vi "InputDriveCommands.vi"(11 "All Joysticks":T3) -> (3 "Drive Command Inputs":T1)   [LabVIEW 2012]
uses:
  Input_All_Joysticks.ctl
  Input_Single_Joystick.ctl
  <vilib>/Rock Robotics/WPI/Joystick/WPI_JoystickButtonState.ctl
  Kinect/KinectInputs.ctl
  Input_Commands_Drive.ctl
panel:
  in  "Kinect Inputs":T2
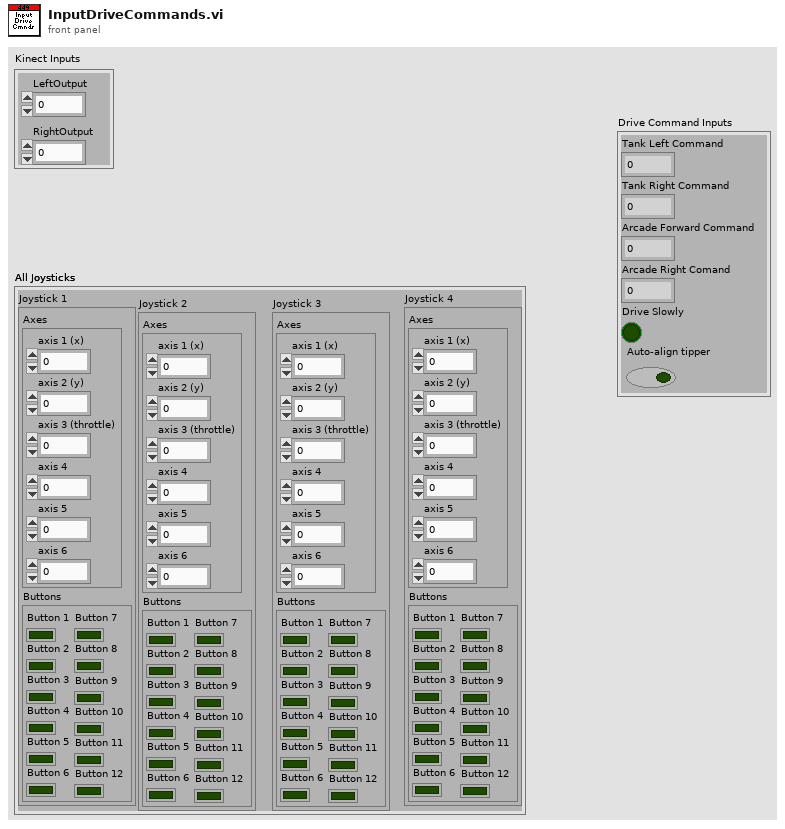
[diagram p1: front panel]
types:
  T1 = typedef "Input_Commands_Drive.ctl" = cluster{"Tank Left Command":dbl, "Tank Right Command":dbl, "Arcade Forward Command":dbl, "Arcade Right Comand":dbl, "Drive Slowly":bool, "Auto-align tipper":bool}
  T2 = typedef "KinectInputs.ctl" = cluster{"LeftOutput":dbl, "RightOutput":dbl}
  T3 = typedef "Input_All_Joysticks.ctl" = cluster{"Joystick 1":T4, "Joystick 2":T4, "Joystick 3":T4, "Joystick 4":T4}
  T4 = typedef "Input_Single_Joystick.ctl" = cluster{"Axes":cluster{"axis 1 (x)":dbl, "axis 2 (y)":dbl, "axis 3 (throttle)":dbl, "axis 4":dbl, "axis 5":dbl, "axis 6":dbl}, "Buttons":T5}
  T5 = typedef "WPI_JoystickButtonState.ctl" = cluster{"Button 1":bool, "Button 2":bool, "Button 3":bool, "Button 4":bool, "Button 5":bool, "Button 6":bool, "Button 7":bool, "Button 8":bool, "Button 9":bool, "Button 10":bool, "Button 11":bool, "Button 12":bool}
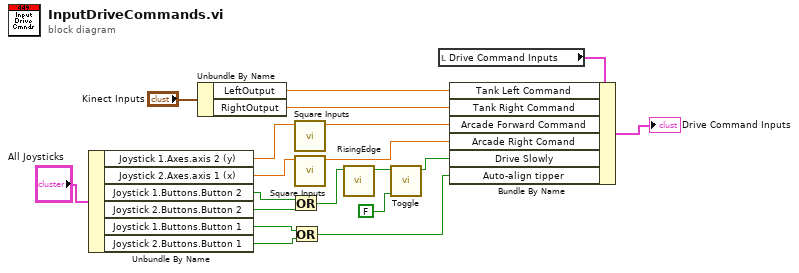
[diagram p0: block diagram]
diagram:
  n1 = Unbundle By Name("All Joysticks") -> ("Joystick 1.Axes.axis 2 (y)"=w17:dbl, "Joystick 2.Axes.axis 1 (x)"=w16:dbl, "Joystick 1.Buttons.Button 2"=w9:bool, "Joystick 2.Buttons.Button 2"=w8:bool, "Joystick 1.Buttons.Button 1"=w3:bool, "Joystick 2.Buttons.Button 1"=w2:bool)
  n2 = Unbundle By Name("Kinect Inputs") -> ("LeftOutput"=w12:dbl, "RightOutput"=w11:dbl)
  n3 = Or(x=w9, y=w8) -> (x .or. y?=w4:bool)
  n4 = Or(x=w3, y=w2) -> (x .or. y?=w1:bool)
  n5 = call "Square Inputs.vi"("Input"=w17) -> ("Squared Value"=w15:dbl)  [unwired: 10 in]
  n6 = call "Square Inputs.vi"("Input"=w16) -> ("Squared Value"=w14:dbl)  [unwired: 10 in]
  n7 = call "RisingEdge.vi"("BooleanIn"=w4) -> ("BooleanOut"=w7:bool)  [unwired: 10 in]
  n8 = call "Toggle.vi"("Initial"=FALSE, "Toggle"=w7) -> ("BoolOut"=w5:bool)  [unwired: 9 in]
  n9 = local read "Drive Command Inputs"() -> (w19:T1)
  n10 = Bundle By Name(cluster=w19, "Tank Left Command"=w12, "Tank Right Command"=w11, "Arcade Forward Command"=w15, "Arcade Right Comand"=w14, "Drive Slowly"=w5, "Auto-align tipper"=w1) -> (→"Drive Command Inputs":T1)
